vi "Autonomous.vi"(11 "Call Context":T7) -> (0 "SubState 2":T2, 1 "Loop 2 Data":T3, 2 "SubState 1":T2, 3 "Loop 1 Data":T4, 4 "Loop 3 Data":T1, 5 "SubState 0":T2=enum."driver control", 6 "SubState 3":T2, 7 "Loop 0 Data":T5, 10 "SubState 4":T6)   [LabVIEW 2013]
uses:
  typedefs/State Machine/subStates.ctl
  <vilib>/Rock Robotics/WPI/DriverStation/WPI_DriverStationDerivedRobotMode.ctl
  typedefs/State Machine/singleUseSubstate.ctl
  typedefs/Loop Datatypes/Loop 0 Datatype.ctl
  typedefs/Loop Datatypes/Loop 1 Datatype.ctl
  typedefs/Loop Datatypes/Loop 2 Datatype.ctl
  typedefs/Loop Datatypes/Loop 3 Datatype.ctl
  typedefs/fg_typedef.ctl
  typedefs/Vision/vision enable.ctl
panel:
  # "Autonomous Loop Data"
  # "Robot Drive"
  # "State Machine Master"
  # "Pickup/Passing Belts"
  # "Pickup/Passing Arm"
  # "Pneumatics"
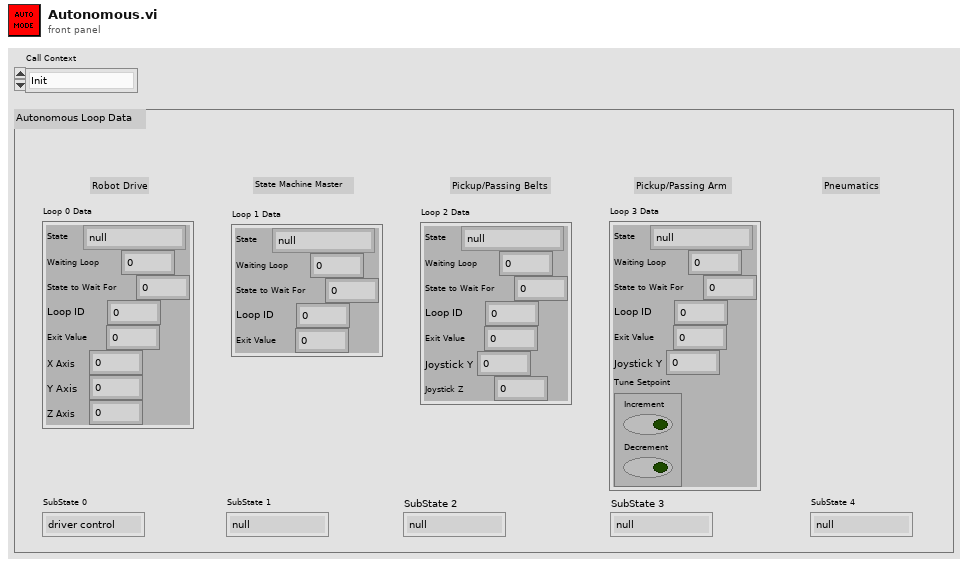
[diagram p1: front panel]
types:
  T1 = typedef "Loop 3 Datatype.ctl" = cluster{"State":T2, "Waiting Loop":i32, "State to Wait For":i32, "Loop ID":i32, "Exit Value":i32, "Joystick Y":dbl, "Tune Setpoint":cluster{"Increment":bool, "Decrement":bool}}
  T2 = typedef "subStates.ctl" = enum16{"null", "wait", "driver control", "auto", "manual override", "hold position", "rotate", "pickup", "pass", "recover pass", "load", "goto shoot", "shoot high goal", "shoot low goal", "cancel arm", "cancel shooter", "end", "test"}
  T3 = typedef "Loop 2 Datatype.ctl" = cluster{"State":T2, "Waiting Loop":i32, "State to Wait For":i32, "Loop ID":i32, "Exit Value":i32, "Joystick Y":dbl, "Joystick Z":dbl}
  T4 = typedef "Loop 1 Datatype.ctl" = cluster{"State":T2, "Waiting Loop":i32, "State to Wait For":i32, "Loop ID":i32, "Exit Value":i32}
  T5 = typedef "Loop 0 Datatype.ctl" = cluster{"State":T2, "Waiting Loop":i32, "State to Wait For":i32, "Loop ID":i32, "Exit Value":i32, "X Axis":dbl, "Y Axis":dbl, "Z Axis":dbl}
  T6 = typedef "singleUseSubstate.ctl" = enum16{"null", "wait", "shift high", "shift low", "extend shooter", "retract shooter", "latch", "unlatch", "end"}
  T7 = typedef "WPI_DriverStationDerivedRobotMode.ctl" = enum16{"Init", "Execute", "Stop"}
  T8 = typedef "vision enable.ctl" = enum16{"Enable", "Disable", "Stop"}
  T9 = typedef "fg_typedef.ctl" = enum16{"Get", "Set"}
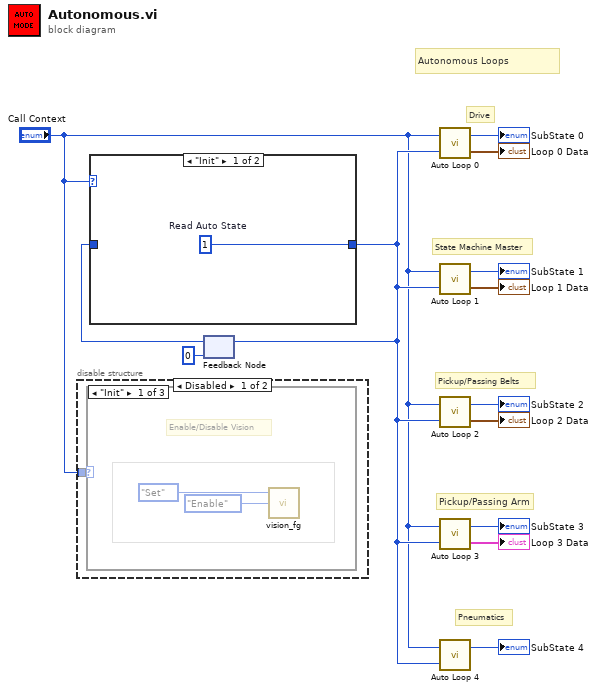
[diagram p0: block diagram]
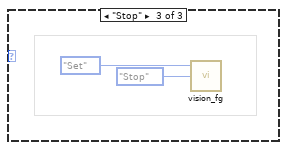
[diagram p3: hidden frame]
diagram:
  # "Autonomous Loops"
  # "Pickup/Passing Arm"
  # "Pickup/Passing Belts"
  # "Pneumatics"
  # "State Machine Master"
  # "Drive"
  n1 = disable-structure shown="Disabled" {
    disable-tunnel: "Call Context" -> [w14 _]
    frame Disabled {
      n2 = case shown="\"Init\"" w14 {
        frame "Init" {
          # "Enable/Disable Vision"
          n3 = call "vision_fg.vi"("Action"=vision_enable."Enable", "Menu"=fg_typedef."Set") -> ()  [unwired: 1 in, 2 out]
        }
        frame "Execute", Default {
        }
        frame "Stop" {
          n4 = call "vision_fg.vi"("Action"=vision_enable."Stop", "Menu"=fg_typedef."Set") -> ()  [unwired: 1 in, 2 out]
        }
      }
    }
    frame Enabled {
    }
  }
  n5 = feedback #1(u8 0 ("Read Auto State")) -> (w2:u8)
  n6 = case shown="\"Init\"" "Call Context" {
    tunnel: [w19 w20] -> w4
    tunnel: w2 -> [_ w20]
    frame "Init" {
      w19 = u8 1  # Read Auto State
    }
    frame "Execute", Default {
    }
  }
  n7 = feedback-in #1(w4) -> ()
  n8 = call "Auto Loop 0.vi"("Auto State"=w4, "Call Context"="Call Context") -> ("Loop 0 Data"=→"Loop 0 Data":T5, "SubState 0"=→"SubState 0":T2)
  n9 = call "Auto Loop 1.vi"("Auto State"=w4, "Call Context"="Call Context") -> ("Loop 1 Data"=→"Loop 1 Data":T4, "SubState 1"=→"SubState 1":T2)
  n10 = call "Auto Loop 2.vi"("Auto State"=w4, "Call Context"="Call Context") -> ("Loop 2 Data"=→"Loop 2 Data":T3, "SubState 2"=→"SubState 2":T2)
  n11 = call "Auto Loop 3.vi"("Auto State"=w4, "Call Context"="Call Context") -> ("Loop 3 Data"=→"Loop 3 Data":T1, "SubState 3"=→"SubState 3":T2)
  n12 = call "Auto Loop 4.vi"("Auto State"=w4, "Call Context"="Call Context") -> ("SubState 5"=→"SubState 4":T6)  [unwired: 1 in]
